vi "타임FGV.vi"(1 "열거형":enum16{"초기화", "카운트", "정지"}(ring)) -> (0 "카운트":u32)   [LabVIEW 2020]
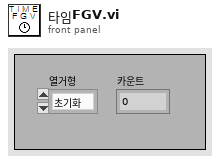
[diagram p1: front panel]
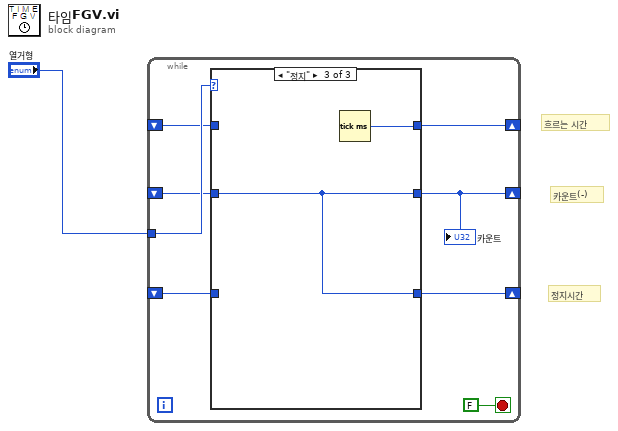
[diagram p0: block diagram]
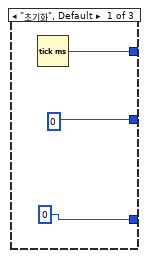
[diagram p2: hidden frame]
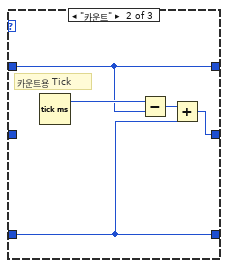
[diagram p3: hidden frame]
diagram:
  # "정지시간"
  # "카운트(-)"
  # "흐르는 시간"
  n1 = while {
    shift-right: [w8] -> _
    shift-left: _ -> [w5]
    shift-right: [w7] -> _
    shift-left: _ -> [w4]
    shift-right: [w6] -> _
    shift-left: _ -> [w3]
    tunnel: "열거형" -> [w9]
    stop <- FALSE stop-if-true
    n2 = case shown="\"정지\"" w9 {
      tunnel: [w12 w15 w19] -> w8
      tunnel: [0 w14 w18] -> w7
      tunnel: [0 w13 w18] -> w6
      tunnel: w5 -> [_ w15 _]
      tunnel: w4 -> [_ _ w18]
      tunnel: w3 -> [_ w13 _]
      frame "초기화", Default {
        n3 = Tick Count (ms)() -> (millisecond timer value=w12:u32)
      }
      frame "카운트" {
        # "카운트용 Tick"
        n4 = Tick Count (ms)() -> (millisecond timer value=w16:u32)
        n5 = Subtract(x=w16, y=w15) -> (x-y=w17:u32)
        n6 = Add(x=w17, y=w13) -> (x+y=w14:u32)
      }
      frame "정지" {
        n7 = Tick Count (ms)() -> (millisecond timer value=w19:u32)
      }
    }
    "카운트" <- w7
  }
